vi "ArmFeedForwardCalculations.vi"(6 "Motor Torque Compensation":dbl[](array[numeric]), 8 "Wrist Pos (deg)":dbl, 9 "Elbow Pos (deg)":dbl, 10 "Shoulder Pos (deg)":dbl) -> (0 "Wrist Power [-1, 1]":dbl, 1 "Elbow Power [-1. 1]":dbl, 2 "Shoulder Power [-1, 1]":dbl)   [LabVIEW 2020]
doc: "Takes in current joint positions and outputs necessary powers to fight gravity"
uses:
  GlobalArm.vi
  GlobalGripper.vi
  <vilib>/robotics/Kinematics/dyn/Gravity Loading (Point).vi
  <vilib>/robotics/Kinematics/NI_Kinematics.lvlib
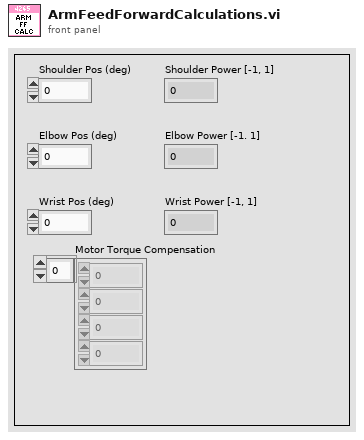
[diagram p1: front panel]
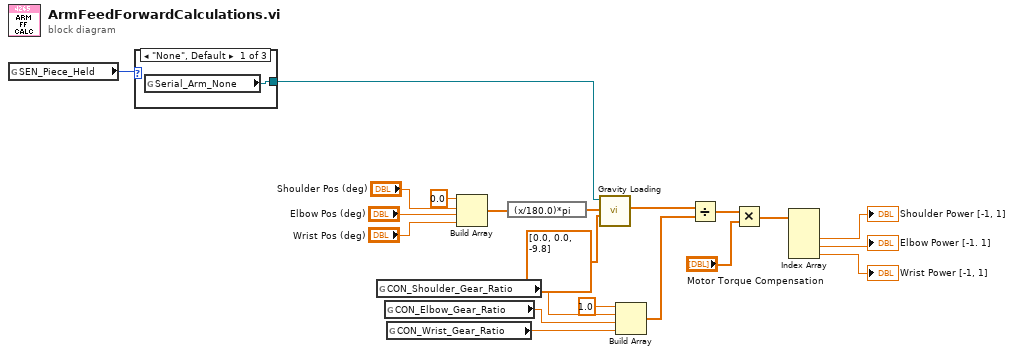
[diagram p0: block diagram]
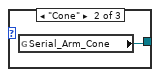
[diagram p2: hidden frame]
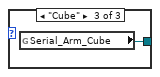
[diagram p3: hidden frame]
diagram:
  n1 = global read "GlobalGripper.vi" "SEN_Piece_Held"() -> (w20:enum16{"None", "Cube", "Cone"})
  n2 = case shown="\"None\", Default" w20 {
    tunnel: [w22 w23 w24] -> w21
    frame "None", Default {
      n3 = global read "GlobalArm.vi" "Serial_Arm_None"() -> (w22:refnum<class "NI_Robotics_Serial Robot Arm.lvclass">)
    }
    frame "Cone" {
      n4 = global read "GlobalArm.vi" "Serial_Arm_Cone"() -> (w23:refnum<class "NI_Robotics_Serial Robot Arm.lvclass">)
    }
    frame "Cube" {
      n5 = global read "GlobalArm.vi" "Serial_Arm_Cube"() -> (w24:refnum<class "NI_Robotics_Serial Robot Arm.lvclass">)
    }
  }
  n6 = global read "GlobalArm.vi" "CON_Shoulder_Gear_Ratio"() -> (w16:dbl)
  n7 = global read "GlobalArm.vi" "CON_Elbow_Gear_Ratio"() -> (w17:dbl)
  n8 = global read "GlobalArm.vi" "CON_Wrist_Gear_Ratio"() -> (w18:dbl)
  n9 = Build Array(0.0 ("element"), "Shoulder Pos (deg)", "Elbow Pos (deg)", "Wrist Pos (deg)") -> (w2:dbl[])
  n10 = expression code="(x/180.0)*pi" ("degrees to radians")(w2) -> (w1:dbl[])
  n11 = call-poly <vilib>:"Gravity Loading.vi"("gravity"=dbl[] [0.0, 0.0, -9.8], "joint positions"=w1, "serial arm in"=w21) -> ("torques"=w9:dbl[])  [unwired: 6 in, 2 out]
  n12 = Build Array(1.0 ("element"), w16, w17, w18) -> (w19:dbl[])
  n13 = Divide(x=w9, y=w19) -> (x/y=w10:dbl[])
  n14 = Multiply(x=w10, y="Motor Torque Compensation") -> (x*y=w11:dbl[])
  n15 = Index Array(array=w11) -> (element #2=→"Shoulder Power [-1, 1]":dbl, element #3=→"Elbow Power [-1. 1]":dbl, element #4=→"Wrist Power [-1, 1]":dbl)  [unwired: 4 in, 1 out]
